vi "Configure Acquisition.vi"(5 "Manual Sensitivity (0.65)":dbl=0.65, 7 "Autotrigger State (T: On)":bool=TRUE, 8 "error in (no error)":errorcluster, 9 "Auto Sensitivity State (T: On)":bool=TRUE, 10 "Low Pass Filter (T: On)":bool=TRUE, 11 "VISA resource name":refnum<visa-resource-name>) -> (0 "error out":errorcluster, 3 "VISA resource name out":refnum<visa-resource-name>)   [LabVIEW 2019, in "Pendulum CNT90.lvlib"]
doc: "Configures the common properties of the counter's channel. Switches on or off the low pass filter on input A, autotrigger, auto sensitivity and sets sesitivity."
uses:
  Pendulum CNT90.lvlib
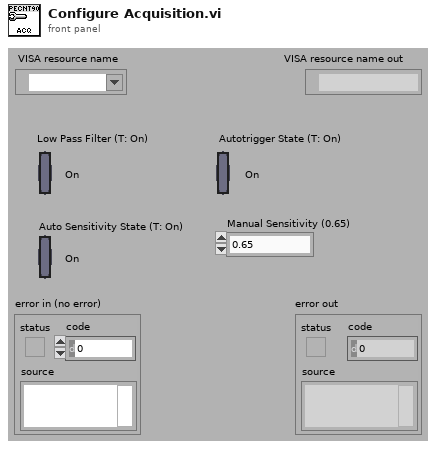
[diagram p1: front panel]
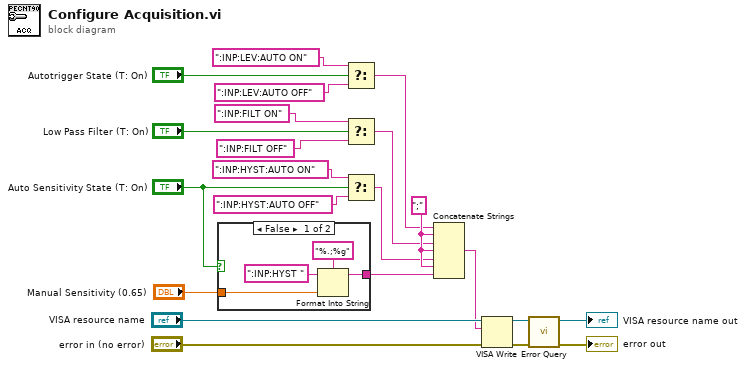
[diagram p0: block diagram]
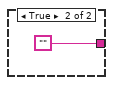
[diagram p2: hidden frame]
diagram:
  w6 = ";"
  n1 = case shown="False" "Auto Sensitivity State (T: On)" {
    tunnel: "Manual Sensitivity (0.65)" -> [w24 _]
    tunnel: [w23 ""] -> w7
    frame False {
      n2 = Format Into String(format string="%.;%g" ("Impedance"), initial string=":INP:HYST " ("Impedance"), w24) -> (resulting string=w23:string)  [unwired: 1 in, 1 out]
    }
    frame True {
    }
  }
  n3 = Select(t=":INP:LEV:AUTO ON" ("string"), s="Autotrigger State (T: On)", f=":INP:LEV:AUTO OFF" ("string")) -> (s? t:f=w5:string)
  n4 = Select(t=":INP:FILT ON" ("string"), s="Low Pass Filter (T: On)", f=":INP:FILT OFF" ("string")) -> (s? t:f=w2:string)
  n5 = Select(t=":INP:HYST:AUTO ON" ("string"), s="Auto Sensitivity State (T: On)", f=":INP:HYST:AUTO OFF" ("string")) -> (s? t:f=w3:string)
  n6 = Concatenate Strings(w5, w6, w2, w6, w3, w6, w7) -> (w4:string)
  n7 = VISA Write(VISA resource name="VISA resource name", write buffer=w4, error in (no error)="error in (no error)") -> (VISA resource name out=w18:refnum<visa-resource-name>, error out=w17:errorcluster)  [unwired: 1 out]
  n8 = call "Error Query.vi"("error in (no error)"=w17, "VISA resource name"=w18) -> ("error out"=→"error out":errorcluster, "VISA resource name out"=→"VISA resource name out":refnum<visa-resource-name>)  [unwired: 6 in, 2 out]
